vi "Shift Rev.vi"(11 "Circular Buffer in":refnum<class "Circular Buffer.lvclass">) -> (3 "Circular Buffer out":refnum<class "Circular Buffer.lvclass">)   [LabVIEW 2021, in "d20.lvlib" / "Circular Buffer.lvclass"]
uses:
  Circular Buffer.lvclass
  Circular Buffer.lvclass/Circular Buffer.ctl
  INode/INode.lvclass
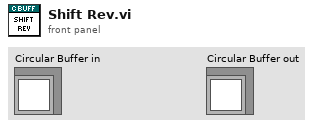
[diagram p1: front panel]
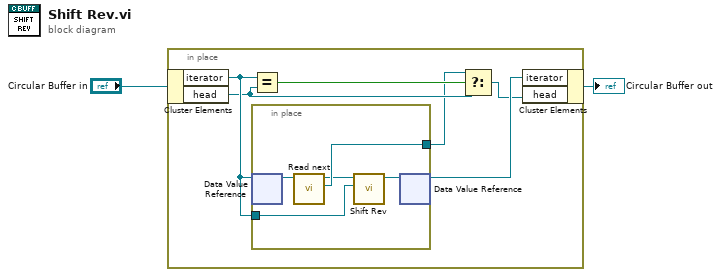
[diagram p0: block diagram]
diagram:
  n1 = in-place {
    n2 = in-place-cluster #1("Circular Buffer in") -> ("iterator"=w8:refnum<data-value>, "head"=w5:refnum<data-value>)
    n3 = Equal?(x=w8, y=w5) -> (x = y?=w6:bool)
    n4 = in-place {
      in-place-border: w8 -> [w13]
      in-place-border: [w12] -> w4
      n5 = in-place-dvr #2(w8) -> (w9:refnum<class "INode.lvclass">)  [unwired: 1 out]
      n6 = call-dynamic "Read next.vi"("Node in"=w9) -> ("next"=w12:refnum<data-value>, "Node out"=w11:refnum<class "INode.lvclass">)  [unwired: 9 in]
      n7 = call-dynamic "Shift Rev.vi"("iterator"=w13, "INode in"=w11) -> ("INode out"=w10:refnum<class "INode.lvclass">)  [unwired: 9 in]
      n8 = in-place-dvr #2(w10) -> (w7:refnum<data-value>)  [unwired: 1 out]
    }
    n9 = Select(t=w4, s=w6, f=w5) -> (s? t:f=w3:refnum<data-value>)
    n10 = in-place-cluster #1("iterator"=w7, "head"=w3) -> (→"Circular Buffer out":refnum<class "Circular Buffer.lvclass">)
  }
